vi "Write Real Wind Sample.vi"(1 "Record ID":u64, 4 "error in":errorcluster, 5 "CSV File Path":path, 7 "Real Wind Sample":T1) -> (0 "error out":errorcluster, 2 "Csv Commit OKK?":bool, 3 "CSV Row Preview":string)   [LabVIEW 2026]
uses:
  Real Wind Sample.ctl
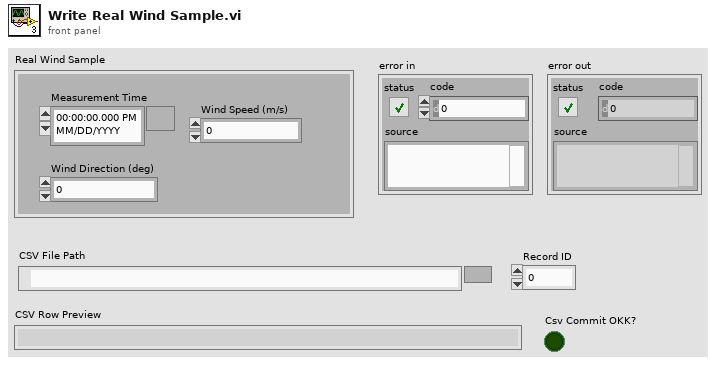
[diagram p1: front panel]
types:
  T1 = typedef "Real Wind Sample.ctl" = cluster{"Measurement Time":timestamp, "Wind Direction (deg)":dbl, "Wind Speed (m/s)":dbl}
  T2 = enum16{"open", "replace", "create", "open or create", "replace or create", "replace or create with confirmation"}
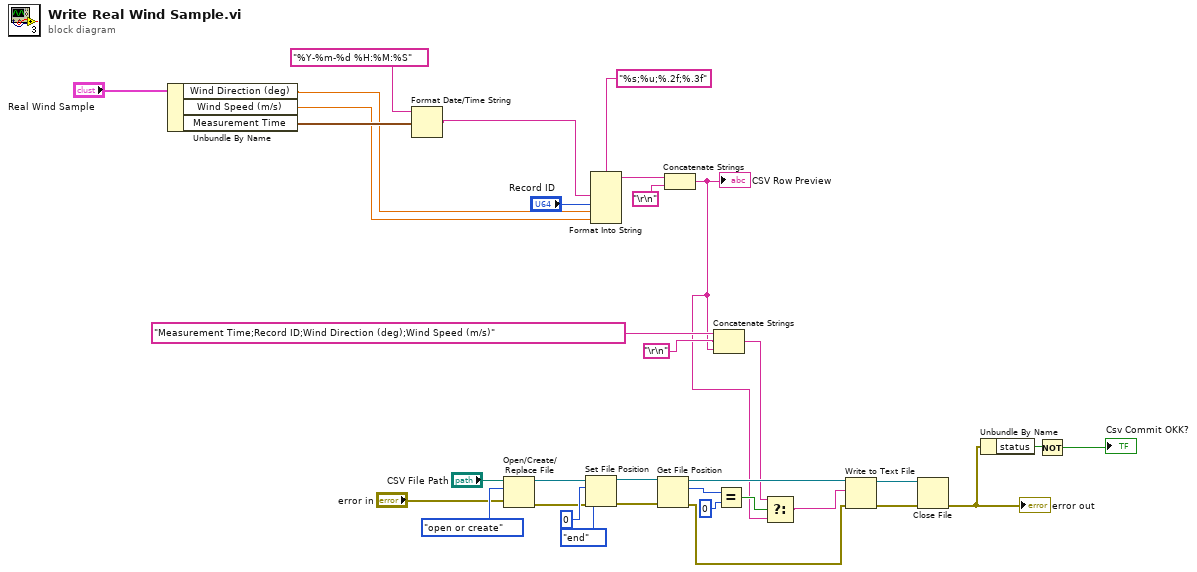
[diagram p0: block diagram]
diagram:
  n1 = Unbundle By Name("Real Wind Sample") -> ("Wind Direction (deg)"=w7:dbl, "Wind Speed (m/s)"=w6:dbl, "Measurement Time"=w34:timestamp)
  n2 = Format Date/Time String(time format string (%c)="%Y-%m-%d %H:%M:%S", seconds (now)=w34) -> (date/time string=w5:string)  [unwired: 1 in]
  n3 = Open/Create/Replace File(file path (use dialog)="CSV File Path", error in="error in", operation (0:open)=T2."open or create") -> (refnum out=w23:refnum<file>, error out=w19:errorcluster)  [unwired: 3 in, 1 out]
  n4 = Set File Position(offset (in bytes) (0)=i64 0, refnum=w23, from (0:start)=enum16{"start", "end", "current"}."end", error in=w19) -> (refnum out=w22:refnum<file>, error out=w18:errorcluster)
  n5 = Format Into String(format string="%s;%u;%.2f;%.3f", w5, "Record ID", w7, w6) -> (resulting string=w31:string)  [unwired: 2 in, 1 out]
  n6 = Get File Position(4:w18, 7:w22) -> (0:w12:errorcluster, 2:w25:i64, 3:w15:refnum<file>)
  n7 = Concatenate Strings(w31, "\r\n") -> (w9:string)
  "CSV Row Preview" <- w9
  n8 = Concatenate Strings("Measurement Time;Record ID;Wind Direction (deg);Wind Speed (m/s)", "\r\n", w9) -> (w14:string)
  n9 = Equal?(x=w25, y=i64 0) -> (x = y?=w16:bool)
  n10 = Select(t=w14, s=w16, f=w9) -> (s? t:f=w13:string)
  n11 = Write to Text File(file (use dialog)=w15, text=w13, error in=w12) -> (refnum out=w21:refnum<file>, error out=w17:errorcluster)  [unwired: 1 in, 1 out]
  n12 = Close File(refnum=w21, error in=w17) -> (error out=w3:errorcluster)  [unwired: 1 out]
  "error out" <- w3
  n13 = Unbundle By Name(w3) -> ("status"=w2:bool)
  n14 = Not(x=w2) -> (.not. x?=→"Csv Commit OKK?":bool)
